vi "timestamp to string (UTC).vi"() -> (8 "date/time string (UTC)":string, 15 "UTC [s]":dbl)   [LabVIEW 2010, in "util.lvlib"]
uses:
  util.lvlib
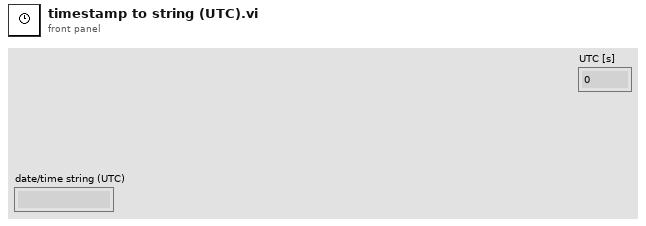
[diagram p1: front panel]
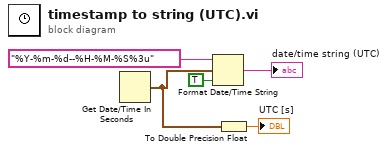
[diagram p0: block diagram]
diagram:
  n1 = Get Date/Time In Seconds() -> (seconds since 1Jan1904=w2:timestamp)
  n2 = Format Date/Time String(time format string (%c)="%Y-%m-%d--%H-%M-%S%3u" ("Zeitformatierungs-String (%c)"), seconds (now)=w2, UTC format=TRUE ("Weltzeit")) -> (date/time string=→"date/time string (UTC)":string)
  n3 = To Double Precision Float(number=w2) -> (double precision float=→"UTC [s]":dbl)
